vi "Calculate Resample Parameters.vi"(9 "Original Frame Size (Samples)":i64=200000, 10 "Original Sample Rate (S/s)":dbl=200000.0, 11 "Sound Format":T1={"channel"=enum."mono", "sample rate (S/s)"=enum."44100", "bits per sample"=enum."16 bit"}) -> (1 "Audio Waveform Init":waveform(dbl), 3 "IQ Waveform Init":waveform(cdb), 4 "Resample Buffer Size (Samp)":i32, 5 "Resample Rate (dt)":dbl)   [LabVIEW 2020]
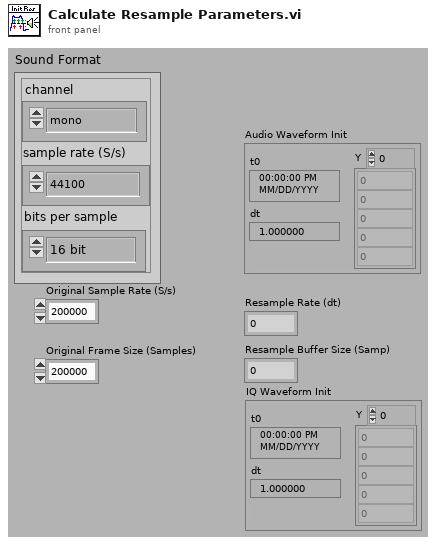
[diagram p1: front panel]
types:
  T1 = cluster{"channel":enum16{"mono", "stereo"}, "sample rate (S/s)":enum16{"11025", "22050", "44100", "8000"}, "bits per sample":enum16{"8 bit", "16 bit"}}
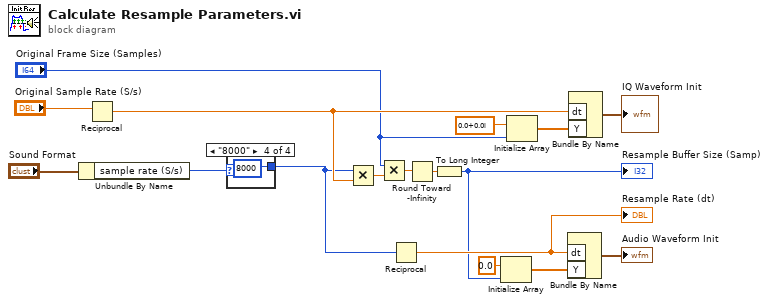
[diagram p0: block diagram]
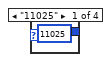
[diagram p2: hidden frame]
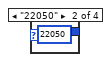
[diagram p3: hidden frame]
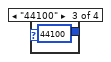
[diagram p4: hidden frame]
diagram:
  n1 = Unbundle By Name("Sound Format") -> ("sample rate (S/s)"=w2:enum16{"11025", "22050", "44100", "8000"})
  n2 = Reciprocal(x="Original Sample Rate (S/s)") -> (1/x=w7:dbl)
  n3 = case shown="\"8000\"" w2 {
    tunnel: [u32 11025 u32 22050 u32 44100 u32 8000] -> w1
    frame "11025" {
    }
    frame "22050" {
    }
    frame "44100" {
    }
    frame "8000" {
    }
  }
  n4 = Multiply(x=w1, y=w7) -> (x*y=w16:dbl)
  n5 = Multiply(x="Original Frame Size (Samples)", y=w16) -> (x*y=w14:dbl)
  n6 = Reciprocal(x=w1) -> (1/x=w11:dbl)
  "Resample Rate (dt)" <- w11
  n7 = Round Toward -Infinity(1:w14) -> (0:w13:dbl)
  n8 = To Long Integer(number=w13) -> (32bit integer=w9:i32)
  "Resample Buffer Size (Samp)" <- w9
  n9 = Initialize Array(0.0 ("element"), w9) -> (w17:dbl[])
  n10 = Initialize Array(cdb 0.0+0.0i, "Original Frame Size (Samples)") -> (w4:cdb[])
  n11 = Bundle By Name("dt"=w11, "Y"=w17) -> (→"Audio Waveform Init":waveform(dbl))  [unwired: 1 in]
  n12 = Bundle By Name("dt"=w7, "Y"=w4) -> (→"IQ Waveform Init":waveform(cdb))  [unwired: 1 in]
